vi "PCO_GetFanControlParameters.vi"(8 "error in (no error)":errorcluster {"code" format="%x"}, 11 "ph":u64) -> (0 "error out":errorcluster {"code" format="%x"}, 1 "wMode":u16, 2 "ErrorMessage":i32 format="%x", 3 "ph out":u64, 5 "wValue":u16)   [LabVIEW 2020, in "SDK.lvlib" / "GeneralCameraControl.lvlib"]
doc: "SC2_SDK_FUNC int WINAPI PCO_GetFanControlParameters(HANDLE hCam, WORD* wMode, WORD* wValue, WORD* wReserved, WORD wNumReserved);"
uses:
  GeneralCameraControl.lvlib
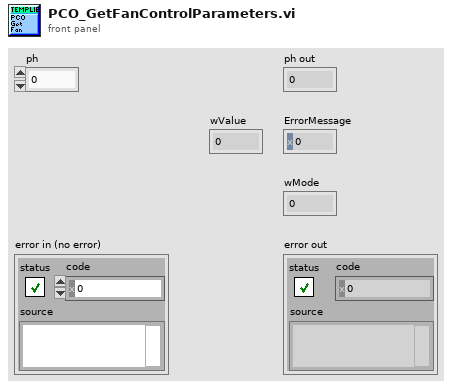
[diagram p1: front panel]
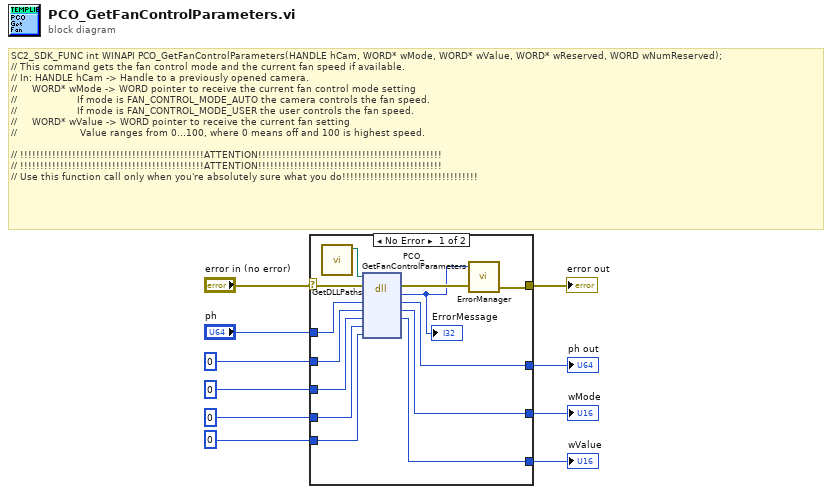
[diagram p0: block diagram]
diagram:
  # "SC2_SDK_FUNC int WINAPI PCO_GetFanControlParameters(HANDLE hCam, WORD* wMode, WORD* wValue, WORD* wReserved, WORD wNumReserved);\n// This command gets the fan control mode and the current fan speed if available.\n// In: HANDLE hCam -> Handle to a previously opened camera.\n//     WORD* wMode -> WORD pointer to receive the current fan control mode setting\n//                    If mode is FAN_CONTROL_MODE_AUTO the camera controls the fan speed.\n//                    If mode is FAN_CONTROL_MODE_USER the user controls the fan speed. \n//     WORD* wValue -> WORD pointer to receive the current fan setting\n//                     Value ranges from 0...100, where 0 means off and 100 is highest speed.\n\n// !!!!!!!!!!!!!!!!!!!!!!!!!!!!!!!!!!!!!!!!!!!!!!ATTENTION!!!!!!!!!!!!!!!!!!!!!!!!!!!!!!!!!!!!!!!!!!!!!!\n// !!!!!!!!!!!!!!!!!!!!!!!!!!!!!!!!!!!!!!!!!!!!!!ATTENTION!!!!!!!!!!!!!!!!!!!!!!!!!!!!!!!!!!!!!!!!!!!!!!\n// Use this function call only when you're absolutely sure what you do!!!!!!!!!!!!!!!!!!!!!!!!!!!!!!!!!!"
  n1 = case shown="No Error" "error in (no error)" {
    selector: "error in (no error)" -> [w15 w27]
    tunnel: "ph" -> [w23 w26]
    tunnel: [w22 w26] -> w9
    tunnel: u16 0 ("wMode") -> [w21 w25]
    tunnel: [w20 w25] -> w7
    tunnel: u16 0 ("wValue") -> [w19 w24]
    tunnel: [w18 w24] -> w5
    tunnel: u16 0 ("wReserved") -> [w17 _]
    tunnel: [w13 w27] -> w3
    tunnel: u16 0 ("wReserved") -> [w16 _]
    frame No Error {
      n2 = call "GetDLLPaths.vi"() -> ("SC2_Cam_Path"=w11:path)  [unwired: 9 in, 2 out]
      n3 = dll-call lib="?" fn="PCO_GetFanControlParameters"(path in=w11, error in=w15, "ph"=w23, "wMode"=w21, "wValue"=w19, "wReserved"=w17, "wNumReserved"=w16) -> (error out=w14:errorcluster, "return type"=w12:i32, "ph"=w22:u64, "wMode"=w20:u16, "wValue"=w18:u16)  [unwired: 3 in, 1 out]
      "ErrorMessage" <- w12
      n4 = call "ErrorManager.vi"("error in (no error)"=w14, "error code"=w12) -> ("error out"=w13:errorcluster)  [unwired: 3 in]
    }
    frame Error {
    }
  }
  "ph out" <- w9
  "wMode" <- w7
  "wValue" <- w5
  "error out" <- w3
